vi "Comparision VI.vi"() -> ()   [LabVIEW 2020]
panel:
  out "x":dbl
  in  "Numeric 2":dbl
  in  "Numeric":dbl
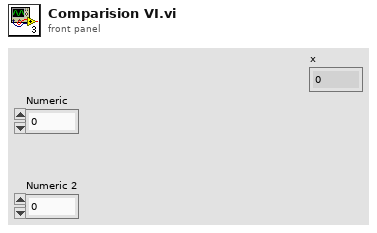
[diagram p1: front panel]
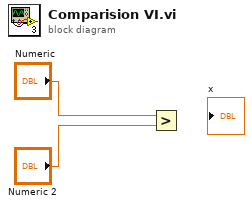
[diagram p0: block diagram]
diagram:
  n1 = Greater?(x="Numeric", y="Numeric 2") -> ()  [unwired: 1 out]
